vi "Array of String_ASCII String To Data.vi"(8 "error in (no error)":errorcluster, 9 "Default":cluster{"String Array":string[]}, 11 "Value":string) -> (0 "error out":errorcluster, 3 "Data":cluster{"String Array":string[]})   [LabVIEW 2010, in "Current Value Table.lvlib"]
doc: "This VI converts data stored on disk as an ascii string into the correct data type. This VI must perform the opposite operation to the DataToASCIIString function."
uses:
  Current Value Table.lvlib
  Errors/Generate Error.vi
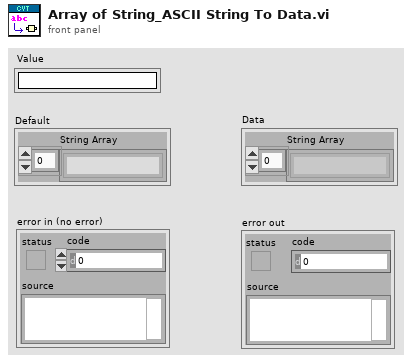
[diagram p1: front panel]
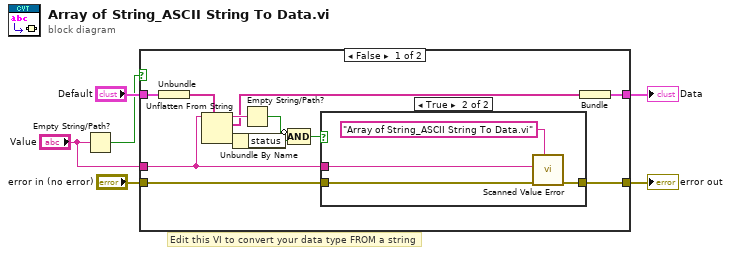
[diagram p0: block diagram]
diagram:
  # "Edit this VI to convert your data type FROM a string"
  n1 = Empty String/Path?(string/path="Value") -> (empty?=w3:bool)
  n2 = case shown="False" w3 {
    tunnel: "Default" -> [w18 w25]
    tunnel: "Value" -> [w8 _]
    tunnel: [w9 w25] -> w1
    tunnel: "error in (no error)" -> [w14 w24]
    tunnel: [w15 w24] -> w5
    frame False {
      n3 = Unbundle(w18) -> ("String Array"=w13:string[])
      n4 = Unflatten From String(type=w13, binary string=w8) -> (rest of the binary string=w11:string, value=w10:string[], error out=w12:errorcluster)  [unwired: 3 in]
      n5 = Unbundle By Name(w12) -> ("status"=w7:bool)
      n6 = Empty String/Path?(string/path=w11) -> (empty?=w17:bool)
      n7 = Compound Arithmetic op=AND(invert w17, w7) -> (w16:bool)
      n8 = case shown="True" w16 {
        tunnel: [w19 w23] -> w15
        tunnel: w14 -> [w19 w22]
        tunnel: w8 -> [_ w21]
        frame False {
        }
        frame True {
          n9 = call "Scanned Value Error.vi"("caller name"="Array of String_ASCII String To Data.vi", "error in (no error)"=w22, "Value"=w21) -> ("error out"=w23:errorcluster)  [unwired: 8 in]
        }
      }
      n10 = Bundle("String Array"=w10) -> (w9:cluster{"String Array":string[]})  [unwired: 1 in]
    }
    frame True {
    }
  }
  "error out" <- w5
  "Data" <- w1
